vi "ABC Find Close.vi"(4 "UART":refnum<vi>, 5 "ComPort":refnum<visa-resource-name>, 6 "Data":refnum<vi>, 7 "DaqTask":refnum<k21>, 8 "ErrIn":errorcluster, 9 "RunWith":cluster{"Steps":i32, "Rates":i32}={"Steps"=400, "Rates"=40}, 10 "Strip":string, 11 "DataIn":dbl[](array[numeric])=[0.0]) -> (0 "ErrOut":errorcluster, 1 "FrontClose":dbl, 3 "DataOut":dbl[](array[numeric]))   [LabVIEW 2020]
uses:
  <userlib>/Amira UART/Public/TypeDefs/AUART StepDir.ctl
  <vilib>/DAQmx/read.llb/DAQmx Read (Digital 1D Bool 1Chan 1Samp).vi
  <vilib>/DAQmx/miscellaneous.llb/DAQmx Fill In Error Info.vi
  <userlib>/Amira UART/Amira UART.lvclass
  <userlib>/KQD LabVIEW User/Serial/Serial.lvlib
panel:
  out "FrontSW":bool
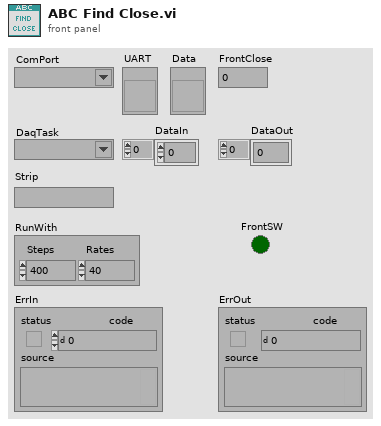
[diagram p1: front panel]
types:
  T1 = typedef "Amira UART.lvclass/AUART StepDir.ctl" = enum16{"", "compress", "decompress"}
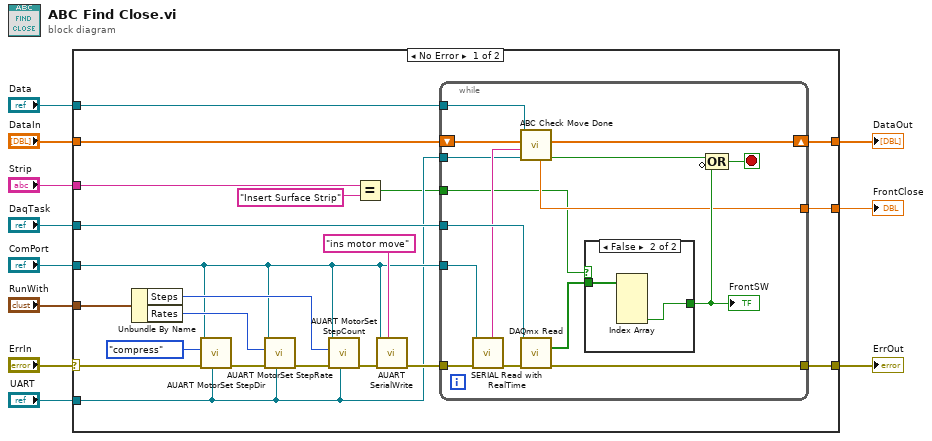
[diagram p0: block diagram]
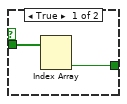
[diagram p2: hidden frame]
diagram:
  n1 = case shown="No Error" "ErrIn" {
    selector: "ErrIn" -> [w28 w53]
    tunnel: "UART" -> [w16 _]
    tunnel: "DaqTask" -> [w32 _]
    tunnel: [w31 w53] -> w9
    tunnel: "DataIn" -> [w30 w54]
    tunnel: [w29 w54] -> w7
    tunnel: "ComPort" -> [w19 _]
    tunnel: "Data" -> [w27 _]
    tunnel: "RunWith" -> [w23 _]
    tunnel: [w15 _] -> w2
    tunnel: "Strip" -> [w14 _]
    frame No Error {
      n2 = Unbundle By Name(w23) -> ("Steps"=w21:i32, "Rates"=w20:i32)
      n3 = call <userlib>:"AUART MotorSet StepDir.vi"("UART"=w16, "ErrIn"=w28, "step_dir"=AUART_StepDir."compress", "Port"=w19) -> ("ErrOut"=w18:errorcluster)  [unwired: 7 in]
      n4 = call <userlib>:"AUART MotorSet StepRate.vi"("UART"=w16, "ErrIn"=w18, "step_rate"=w20, "Port"=w19) -> ("ErrOut"=w17:errorcluster)  [unwired: 7 in]
      n5 = call <userlib>:"AUART MotorSet StepCount.vi"("UART"=w16, "ErrIn"=w17, "step_count"=w21, "Port"=w19) -> ("ErrOut"=w26:errorcluster)  [unwired: 7 in]
      n6 = Equal?(x=w14, y="Insert Surface Strip") -> (x = y?=w12:bool)
      n7 = call <userlib>:"AUART SerialWrite.vi"("Cmd"="ins motor move", "ErrIn"=w26, "Port"=w19) -> ("ErrOut"=w25:errorcluster)  [unwired: 7 in, 1 out]
      n8 = while {
        tunnel: w32 -> [w47]
        tunnel: w27 -> [w41]
        tunnel: w19 -> [w46]
        shift-right: [w38] -> w29
        shift-left: w30 -> [w42]
        tunnel: w25 -> [w45]
        tunnel: [w43] -> w31
        tunnel: w16 -> [w39]
        tunnel: [w34] -> w15
        tunnel: w12 -> [w33]
        stop <- w37 stop-if-true
        n9 = call <userlib>:"SERIAL Read with RealTime.vi"("ErrIn"=w45, "PortIn"=w46) -> ("ErrOut"=w44:errorcluster, "Response"=w40:string)  [unwired: 7 in, 1 out]
        n10 = call "ABC Check Move Done.vi"("UART"=w39, "Response"=w40, "DataIn"=w42, "Data"=w41) -> ("Done"=w36:bool, "DataOut"=w38:dbl[], "Position"=w34:dbl)  [unwired: 5 in]
        n11 = call-poly <vilib>:"DAQmx Read.vi"("task/channels in"=w47, "error in"=w44) -> ("data"=w48:bool[], "error out"=w43:errorcluster)  [unwired: 11 in, 1 out]
        n12 = case shown="False" w33 {
          tunnel: w48 -> [w50 w52]
          tunnel: [w49 w51] -> w35
          frame True {
            n13 = Index Array(array=w50) -> (element #2=w49:bool)  [unwired: 2 in, 1 out]
          }
          frame False {
            n14 = Index Array(array=w52) -> (element #4=w51:bool)  [unwired: 4 in, 3 out]
          }
        }
        "FrontSW" <- w35
        n15 = Compound Arithmetic op=OR(w36, invert w35) -> (w37:bool)
      }
    }
    frame Error {
    }
  }
  "ErrOut" <- w9
  "DataOut" <- w7
  "FrontClose" <- w2
